vi "auton selector.vi"() -> ()   [LabVIEW 2014]
uses:
  <vilib>/Rock Robotics/WPI/Joystick/WPI_JoystickGetSetRefNum.vi
  Robot Global Data.vi
panel:
  out "selected file":string
  out "size":i64
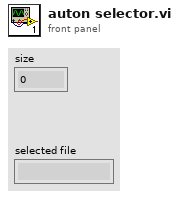
[diagram p1: front panel]
types:
  T1 = typedef "WPI_JoystickDevRef.ctl" = cluster{"Device":T2}
  T2 = typedef "WPI_JoystickDeviceEnum.ctl" = enum16{"USB 0", "USB 1", "USB 2", "USB 3", "USB 4", "USB 5"}
  T3 = cluster{"Buttons[0]":bool, "Buttons[1]":bool, "Buttons[2]":bool, "Buttons[3]":bool, "Buttons[4]":bool, "Buttons[5]":bool, "Buttons[6]":bool, "Buttons[7]":bool, "Buttons[8]":bool}
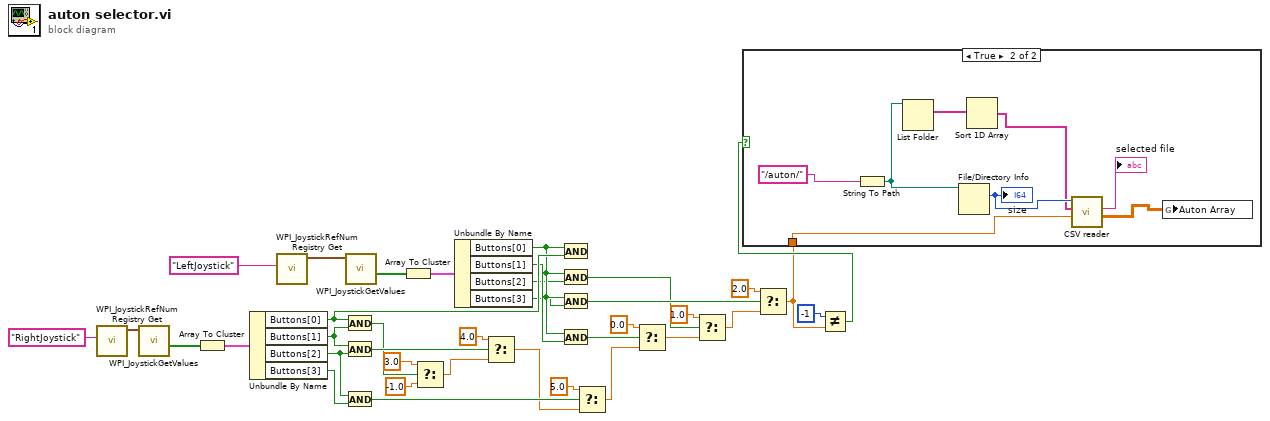
[diagram p0: block diagram]
diagram:
  n1 = call <vilib>:"WPI_JoystickRefNum Registry Get.vi"("refnum name"="RightJoystick") -> ("JoystickDevRef"=w14:T1)  [unwired: 9 in, 1 out]
  n2 = call <vilib>:"WPI_JoystickGetValues.vi"("JoystickDevRef"=w14) -> ("Buttons"=w13:bool[])  [unwired: 6 in, 4 out]
  n3 = Array To Cluster(array=w13) -> (cluster=w12:T3)
  n4 = Unbundle By Name(w12) -> ("Buttons[0]"=w11:bool, "Buttons[1]"=w10:bool, "Buttons[2]"=w9:bool, "Buttons[3]"=w8:bool)
  n5 = call <vilib>:"WPI_JoystickRefNum Registry Get.vi"("refnum name"="LeftJoystick") -> ("JoystickDevRef"=w17:T1)  [unwired: 9 in, 1 out]
  n6 = And(x=w11, y=w10) -> (x .and. y?=w20:bool)
  n7 = And(x=w10, y=w9) -> (x .and. y?=w23:bool)
  n8 = And(x=w9, y=w8) -> (x .and. y?=w28:bool)
  n9 = call <vilib>:"WPI_JoystickGetValues.vi"("JoystickDevRef"=w17) -> ("Buttons"=w15:bool[])  [unwired: 6 in, 4 out]
  n10 = Array To Cluster(array=w15) -> (cluster=w7:T3)
  n11 = Select(t=3.0, s=w20, f=-1.0) -> (s? t:f=w24:dbl)
  n12 = Unbundle By Name(w7) -> ("Buttons[0]"=w6:bool, "Buttons[1]"=w5:bool, "Buttons[2]"=w4:bool, "Buttons[3]"=w3:bool)
  n13 = Select(t=4.0, s=w23, f=w24) -> (s? t:f=w26:dbl)
  n14 = And(x=w6, y=w11) -> ()  [unwired: 1 out]
  n15 = And(x=w6, y=w4) -> (x .and. y?=w33:bool)
  n16 = And(x=w6, y=w3) -> (x .and. y?=w36:bool)
  n17 = And(x=w6, y=w5) -> (x .and. y?=w35:bool)
  n18 = Select(t=5.0, s=w28, f=w26) -> (s? t:f=w37:dbl)
  n19 = Select(t=0.0, s=w35, f=w37) -> (s? t:f=w32:dbl)
  n20 = Select(t=1.0, s=w33, f=w32) -> (s? t:f=w30:dbl)
  n21 = Select(t=2.0, s=w36, f=w30) -> (s? t:f=w1:dbl)
  n22 = Not Equal?(x=-1, y=w1) -> (x != y?=w2:bool)
  n23 = case shown="True" w2 {
    tunnel: w1 -> [_ w40]
    frame False {
    }
    frame True {
      n24 = String To Path(string="/auton/") -> (path=w44:path)
      n25 = List Folder(path=w44) -> (filenames=w43:string[])  [unwired: 3 in, 3 out]
      n26 = File/Directory Info(path=w44) -> (size=w42:i64)  [unwired: 1 in, 6 out]
      "size" <- w42
      n27 = Sort 1D Array(array=w43) -> (sorted array=w41:string[])
      n28 = call "CSV reader.vi"("x"=w40, "Array"=w41, "Number CSV"=w42) -> ("Auton Array"=w38:dbl[][], "File Selected"=→"selected file":string)  [unwired: 7 in]
      n29 = global write "Robot Global Data.vi" "Auton Array"(w38) -> ()
    }
  }
